vi "Get Gen Control Pos Info.vi"(3 "error in":errorcluster, 5 "Ctl Refnum":refnum<vi>) -> (0 "error out":errorcluster, 1 "Pos Info":T1, 2 "Ctl Refnum Out":refnum<vi>)   [LabVIEW 2024, in "EQMF.lvlib" / "Controls.lvlib"]
uses:
  Controls.lvlib
  Resize/Resize, Object Position Info.ctl
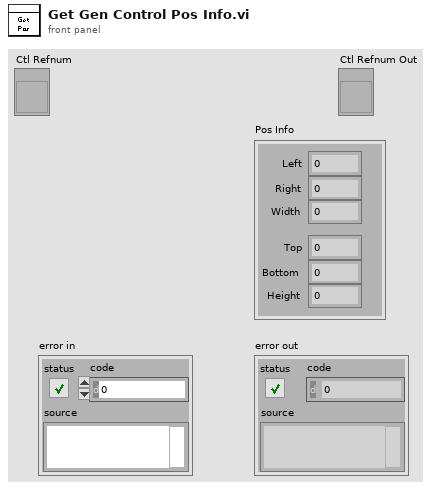
[diagram p1: front panel]
types:
  T1 = typedef "EQMF.lvlib/Controls.lvlib/Resize, Object Position Info.ctl" = cluster{"Left":i32, "Right":i32, "Width":i32, "Top":i32, "Bottom":i32, "Height":i32}
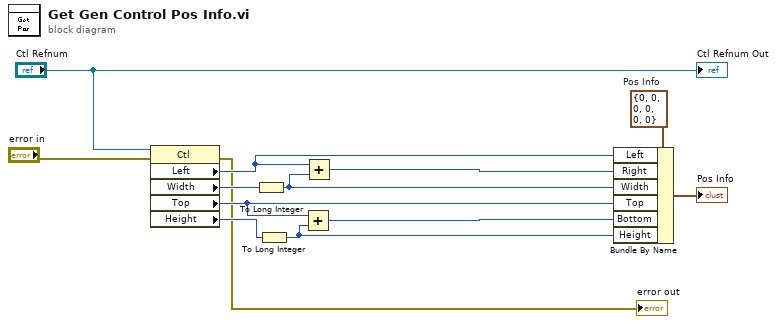
[diagram p0: block diagram]
diagram:
  w13 = T1 {"Left"=0, "Right"=0, "Width"=0, "Top"=0, "Bottom"=0, "Height"=0}  # Pos Info
  n1 = property on="Property Node" class="Ctl"(reference="Ctl Refnum", error in="error in") -> (error out=→"error out":errorcluster, "Left"=w11:i32, "Width"=w4:u32, "Top"=w8:i32, "Height"=w5:u32)  [unwired: 1 out]
  n2 = To Long Integer(number=w4) -> (32bit integer=w9:i32)
  n3 = To Long Integer(number=w5) -> (32bit integer=w6:i32)
  n4 = Add(x=w8, y=w6) -> (x+y=w7:i32)
  n5 = Add(x=w11, y=w9) -> (x+y=w10:i32)
  n6 = Bundle By Name(cluster=w13, "Left"=w11, "Right"=w10, "Width"=w9, "Top"=w8, "Bottom"=w7, "Height"=w6) -> (→"Pos Info":T1)
  "Ctl Refnum Out" <- "Ctl Refnum"
